vi "Modbus Data Accumulator.vi"(10 "Modbus Data":cluster{"Control Name":string, "Value":dbl}[](array[cluster]), 11 "Accumulated Data":string[][](array[string])) -> (3 "Accumulated Data Out":string[][](array[string]))   [LabVIEW 2019]
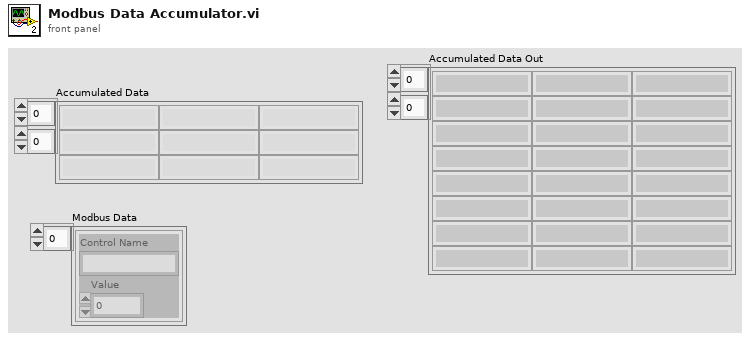
[diagram p1: front panel]
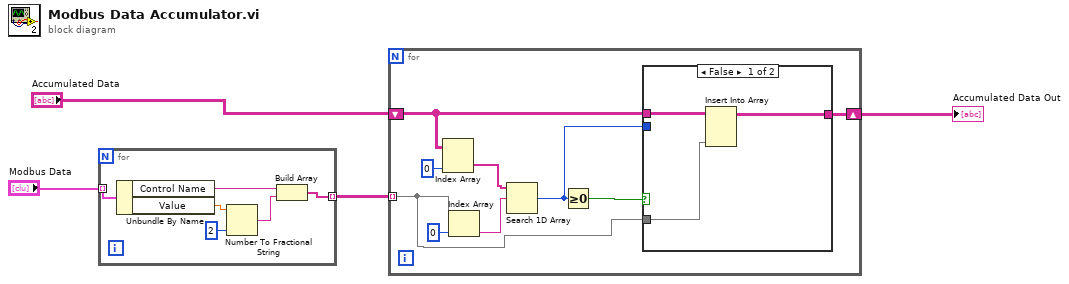
[diagram p0: block diagram]
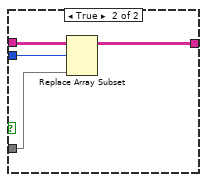
[diagram p2: hidden frame]
diagram:
  n1 = for {
    tunnel: "Modbus Data" -> [w10] mode=indexing
    tunnel: [w5] -> w2 mode=indexing
    n2 = Unbundle By Name(w10) -> ("Control Name"=w6:string, "Value"=w9:dbl)
    n3 = Number To Fractional String(number=w9, precision (6)=i16 2) -> (F-format string=w7:string)  [unwired: 2 in]
    n4 = Build Array(w6, w7) -> (w5:string[])
  }
  n5 = for {
    tunnel: w2 -> [w13] mode=indexing
    shift-right: [w12] -> w1
    shift-left: "Accumulated Data" -> [w15]
    n6 = Index Array(array=w15, index (col)=0 ("disabled index (col)")) -> (element=w17:string[])  [unwired: 1 in]
    n7 = Index Array(array=w13, index=0) -> (element=w18:string)
    n8 = Search 1D Array(1D array=w17, element=w18) -> (index of element=w14:i32)  [unwired: 1 in]
    n9 = Greater Or Equal To 0?(x=w14) -> (x >= 0?=w16:bool)
    n10 = case shown="False" w16 {
      tunnel: w15 -> [w22 w26]
      tunnel: w14 -> [_ w25]
      tunnel: w13 -> [w20 w24]
      tunnel: [w21 w23] -> w12
      frame False {
        n11 = Insert Into Array(array=w22, new element=w20) -> (w21:string[][])  [unwired: 2 in]
      }
      frame True {
        n12 = Replace Array Subset(array=w26, new element=w24, index (row)=w25) -> (w23:string[][])  [unwired: 1 in]
      }
    }
  }
  "Accumulated Data Out" <- w1
